vi "Process.vi"() -> ()   [LabVIEW 2021, in "Launcher Actor.lvclass"]
uses:
  Launcher Actor.lvclass
  Main Controller/API/Main Controller Actor API.lvclass
  Launcher Actor.lvclass/Launcher Actor.ctl
  Glyph.ctl
  Launcher Message.ctl
  Re-use Libraries/Minimal Actor Framework/Messaging/Message/Message.lvclass
  Re-use Libraries/Minimal Actor Framework/Actors/Base Actor/Actor/Front Panel State.ctl
  Re-use Libraries/Minimal Actor Framework/Actors/Base Actor/Actor/Actor.lvclass
  Globals.vi
panel:
  out "Glyph":T1
  out "Message":string="Loading main application, please wait..."
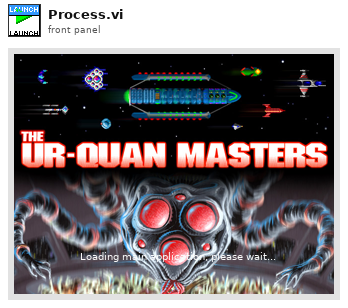
[diagram p1: front panel]
types:
  T1 = typedef "Launcher Actor.lvclass/Glyph.ctl" = u16
  T2 = typedef "Launcher Actor.lvclass/Launcher Message.ctl" = cluster{"Message":string, "Glyph":T1}
  T3 = typedef "Actor.lvclass/Front Panel State.ctl" = enum32{"Invalid", "Standard", "Closed", "Hidden", "Minimized", "Maximized"}
  T4 = enum32{"Invalid", "Standard", "Closed", "Hidden", "Minimized", "Maximized"}
  T5 = enum32{"invalid app kind", "Development System", "Run Time System", "Student Edition", "Embedded LabVIEW", "Evaluation", "Custom"}
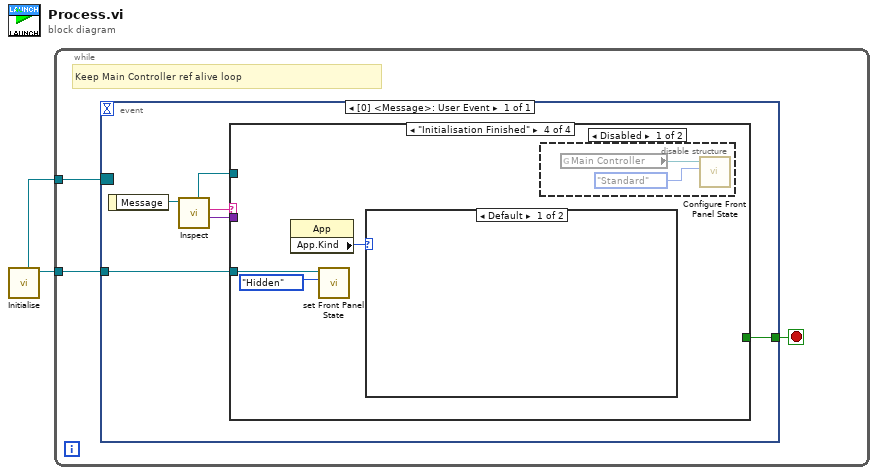
[diagram p0: block diagram]
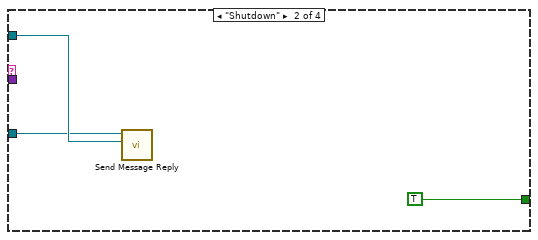
[diagram p3: hidden frame]
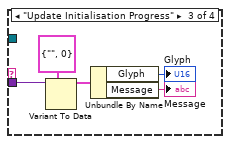
[diagram p4: hidden frame]
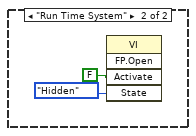
[diagram p6: hidden frame]
diagram:
  n1 = call "Initialise.vi"() -> ("Launcher Actor out"=w2:refnum<class "Launcher Actor.lvclass">, "Actor"=w1:refnum<event-registration>)  [unwired: 9 in, 1 out]
  n2 = while {
    tunnel: w1 -> [w5]
    tunnel: w2 -> [w3]
    stop <- w4 stop-if-true
    # "Keep Main Controller ref alive loop"
    n3 = event shown="[0] <Message>: User Event" {
      selector: w5 -> [_]
      dyn-events: _ -> [_]
      timeout: _ -> [_]
      tunnel: [w8] -> w4
      tunnel: w3 -> [w7]
      event User Event {
        n4 = event-data() -> ("Message"=w11:refnum<class "Message.lvclass">)  [unwired: 1 in]
        n5 = call "Inspect.vi"("Message in"=w11) -> ("Data"=w9:variant, "Name"=w10:string, "Reply Channel"=w6:refnum<notifier>)  [unwired: 6 in, 2 out]
        n6 = case shown="\"Initialisation Finished\"" w10 {
          tunnel: [_ TRUE _ _] -> w8
          tunnel: w9 -> [_ _ w19 _]
          tunnel: w7 -> [_ w12 _ w21]
          tunnel: w6 -> [_ w13 _ _]
          frame Default {
          }
          frame "Shutdown" {
            n7 = call-dynamic "Send Message Reply.vi"("Reply Channel"=w13, "Actor in"=w12) -> ()  [unwired: 8 in, 2 out]
          }
          frame "Update Initialisation Progress" {
            n8 = Variant To Data(type=T2 {"Message"="", "Glyph"=0} ("State Information"), Variant=w19) -> (data=w17:T2)  [unwired: 1 in, 1 out]
            n9 = Unbundle By Name(w17) -> ("Glyph"=→"Glyph":T1, "Message"=→"Message":string)
          }
          frame "Initialisation Finished" {
            n10 = property class="App"() -> ("App.Kind"=w22:T5)  [unwired: 2 in, 2 out]
            n11 = call-dynamic "set Front Panel State.vi"("Front Panel State"=Front_Panel_State."Hidden", "Actor in"=w21) -> ()  [unwired: 8 in, 2 out]
            n12 = case shown="Default" w22 {
              frame Default {
              }
              frame "Run Time System" {
                n13 = invoke class="VI" method="FP.Open"("Activate"=FALSE ("Activate?"), "State"=T4."Hidden") -> ()  [unwired: 3 in, 5 out]
              }
            }
            n14 = disable-structure shown="Disabled" {
              frame Disabled {
                n15 = global read "Globals.vi" "Main Controller"() -> (w24:refnum<class "Main Controller Actor API.lvclass">)
                n16 = call-dynamic "Configure Front Panel State.vi"("Front Panel State"=Front_Panel_State."Standard", "Actor API in"=w24) -> ()  [unwired: 9 in, 1 out]
              }
              frame Enabled {
              }
            }
          }
        }
      }
    }
  }
